vi "MainGUI.vi"(8 "ErrorIn":errorcluster, 11 "Car:Car in":refnum<class "Car.lvclass">) -> ()   [LabVIEW 2021, in "Car.lvlib" / "Car.lvclass"]
uses:
  Car.lvclass
  C:/Localdata/Projects/TriekselSoft/TriekselsoftApplicationFramework/Source/.Externals/Library_YAF/YActor/YActor.lvclass
  Car_UiCallBackEvents.ctl
  Car_ClassCast.vi
  Car.lvclass/Car.ctl
  Source/.Externals/Library_YAF/YActor/YActor.lvclass
  C:/Localdata/Projects/TriekselSoft/TriekselsoftApplicationFramework/Source/.Externals/Library_YAF/YAFTAF/YAFTAF.lvclass
  C:/Localdata/Projects/TriekselSoft/TriekselsoftApplicationFramework/Source/.Externals/Interface_UserInterface_IFrontPanel/IFrontPanel/IFrontPanel.lvclass
  C:/Localdata/Projects/TriekselSoft/TriekselsoftApplicationFramework/Source/.Externals/Interface_TAF_IInterface/IInterface/IInterface.lvclass
  C:/Localdata/Projects/TriekselSoft/TriekselsoftApplicationFramework/Source/.Externals/Interface_Object_ICreateDestroy/ICreateDestroy/ICreateDestroy.lvclass
  C:/Localdata/Projects/TriekselSoft/TriekselsoftApplicationFramework/Source/.Externals/Interface_Object_IPersistentData/IPersistentData/IPersistentData.lvclass
  C:/Localdata/Projects/TriekselSoft/TriekselsoftApplicationFramework/Source/.Externals/Interface_TAF_ITAFObject/ITAFObject/ITAFObject.lvclass
  C:/Localdata/Projects/TriekselSoft/TriekselsoftApplicationFramework/Documentation/Project Documentation/ExampleCode/Car/Car.lvclass
panel:
  out "L_busy":i32
types:
  T1 = typedef "Car.lvlib/Car.lvclass/Car_UiCallBackEvents.ctl" = enum16{"Default", "PersistentDataUpdated"}
  T2 = cluster{"Event":string, "This":refnum<class>, "Data":variant}
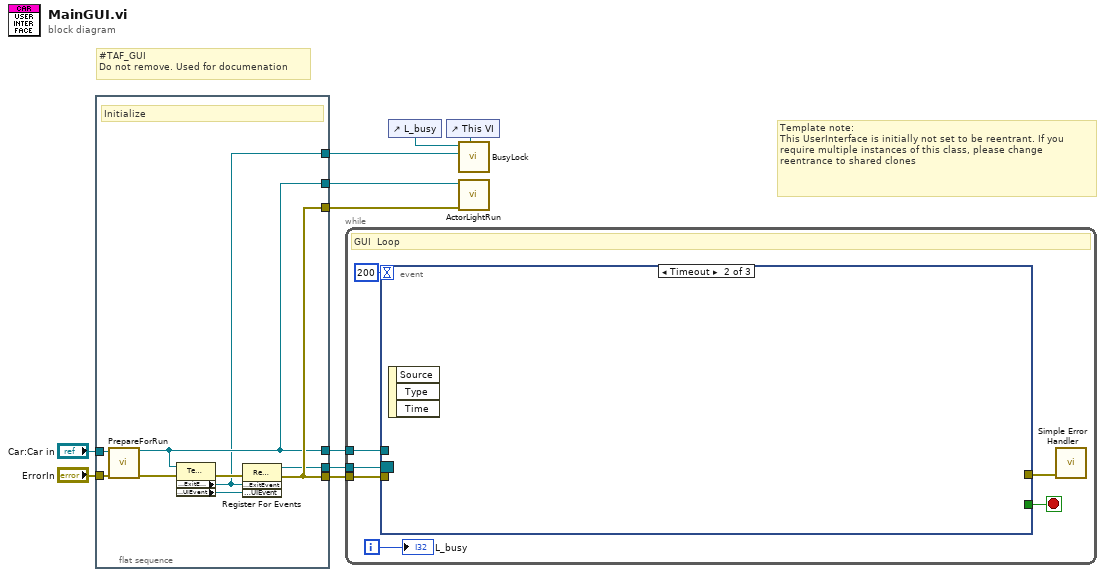
[diagram p0: block diagram]
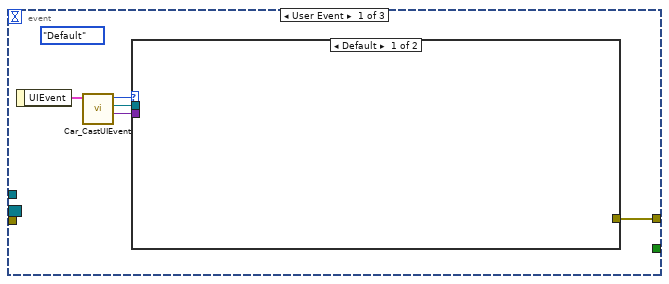
[diagram p2: hidden frame]
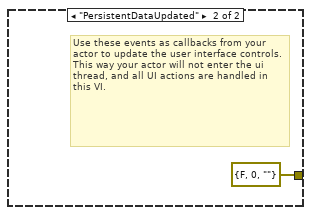
[diagram p3: hidden frame]
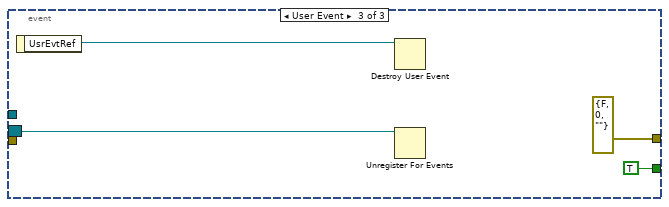
[diagram p4: hidden frame]
diagram:
  # "#TAF_GUI\nDo not remove. Used for documenation"
  # "Template note:\nThis UserInterface is initially not set to be reentrant. If you require multiple instances of this class, please change reentrance to shared clones"
  n1 = flat-sequence {
    tunnel: "ErrorIn" -> [w19]
    tunnel: "Car:Car in" -> [w15]
    tunnel: [w14] -> w6
    tunnel: [w11] -> w3
    tunnel: [w13] -> w1
    tunnel: [w16] -> w9
    tunnel: [w13] -> w2
    tunnel: [w16] -> w8
    frame #0 {
      # "Initialize"
      n2 = call-dynamic "PrepareForRun.vi"("ErrorIn"=w19, "YActorIn"=w15) -> ("ErrorOut"=w17:errorcluster, "YActorOut"=w13:refnum<class "Car.lvclass">)  [unwired: 8 in]
      n3 = property class="TemplateGUITAF"(reference=w13, error in=w17) -> (error out=w18:errorcluster, "properties:ExitEvent"=w11:refnum<user-event>, "properties:UIEvent"=w12:refnum<user-event>)  [unwired: 1 out]
      n4 = register-events(error in=w18, w11, w12) -> (reference out=w14:refnum<event-registration>, error out=w16:errorcluster)  [unwired: 1 in]
    }
  }
  n5 = while {
    tunnel: w9 -> [w26]
    tunnel: w6 -> [w23]
    tunnel: w1 -> [w20]
    i -> [w22]
    stop <- w24 stop-if-true
    # "GUI  Loop"
    n6 = event shown="[1] Timeout" {
      selector: w23 -> [_ _ w34]
      dyn-events: _ -> [_ _ _]
      timeout: 200 -> [_ _ _]
      tunnel: w26 -> [_ _ _]
      tunnel: [_ _ TRUE] -> w24
      tunnel: [w31 _ errorcluster {"status"=FALSE, "code"=0, "source"=""} ("error constant")] -> w25
      tunnel: w20 -> [_ _ _]
      event User Event {
        (unwired) Car_UiCallBackEvents."Default" ("UiEventNames")
        n7 = event-data() -> ("UIEvent"=w30:T2)  [unwired: 1 in]
        n8 = call "Car_CastUIEvent.vi"("UIEvent"=w30) -> ("Data"=w27:variant, "ApplicationGUIOut"=w28:refnum<class "Car.lvclass">, "UiEventNames"=w29:T1)  [unwired: 8 in]
        n9 = case shown="Default" w29 {
          tunnel: w28 -> [_ _]
          tunnel: w27 -> [_ _]
          tunnel: [_ errorcluster {"status"=FALSE, "code"=0, "source"=""} ("ErrorOut")] -> w31
          frame Default {
          }
          frame "PersistentDataUpdated" {
            # "Use these events as callbacks from your actor to update the user interface controls. This way your actor will not enter the ui thread, and all UI actions are handled in this VI."
          }
        }
      }
      event Timeout {
        n10 = event-data() -> ()  [unwired: 1 in, 3 out]
      }
      event User Event {
        n11 = event-data() -> ("UsrEvtRef"=w33:refnum<user-event>)  [unwired: 1 in]
        n12 = Destroy User Event(user event=w33) -> ()  [unwired: 1 in, 1 out]
        n13 = Unregister For Events(event registration refnum=w34) -> ()  [unwired: 1 in, 1 out]
      }
    }
    n14 = call <vilib>:"Simple Error Handler.vi"("error in (no error)"=w25) -> ()  [unwired: 4 in, 5 out]
    "L_busy" <- w22
  }
  n15 = control-ref of="L_busy"() -> (w5:refnum<vi>)
  n16 = control-ref of="This VI"() -> (w4:refnum<vi>)
  n17 = call "BusyLock.vi"("BusyLock"=w4, "ExitEvent"=w3, "Counter"=w5) -> ()  [unwired: 9 in]
  n18 = call "ActorLightRun.vi"("ErrorIn"=w8, "YActorIn"=w2) -> ()  [unwired: 8 in, 2 out]
